vi "FTW-Logger-Construct.vi"(0 "Initialization Sequence":string, 5 "Logger Configuration":string, 11 "error in":errorcluster) -> (4 "FTW Logger":refnum<class "FTW-Logger-Instance.lvclass">, 6 "Incoming Requests":refnum<event-registration>, 15 "error out":errorcluster)   [LabVIEW 2013, in "FTW-Logger-Instance.lvclass"]
uses:
  FTW-Logger-Instance.lvclass
  request/FTW-Request.lvclass
  time/FTW-Time-DisplayFormat-Timestamp.ctl
  FTW-Logger-Instance.lvclass/FTW-Logger-Instance.ctl
  reflection/FTW-Reflection-Type.vi
  json/lib/FTW-JSON-Core-LibraryFilepath.vi
  json/lib/FTW-JSON-Core-GetFlattenedValue.vi
  json/lib/FTW-JSON-Core-LibraryError.vi
  json/FTW-JSON-Deserialize/FTW-JSON-Deserialize.xnode
panel:
  # "Inputs"
  # "Outputs"
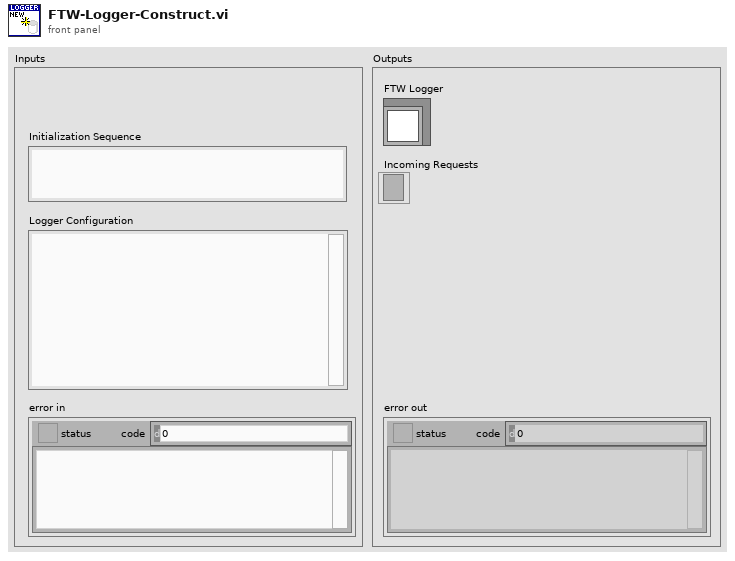
[diagram p1: front panel]
types:
  T1 = typedef "FTW-Time-DisplayFormat-Timestamp.ctl" = enum16{"YYYY-MM-DDT00:00:00.000Z (ISO-8601)", "YYYY-MM-DDT00-00-00Z (Simple ISO-8601)", "YYYY-MM-DD"}
  T2 = cluster{"LoggerDirectory":path, "LoggerDiskThrashDelay":u32, "LoggerName":string, "ApplicationName":string}
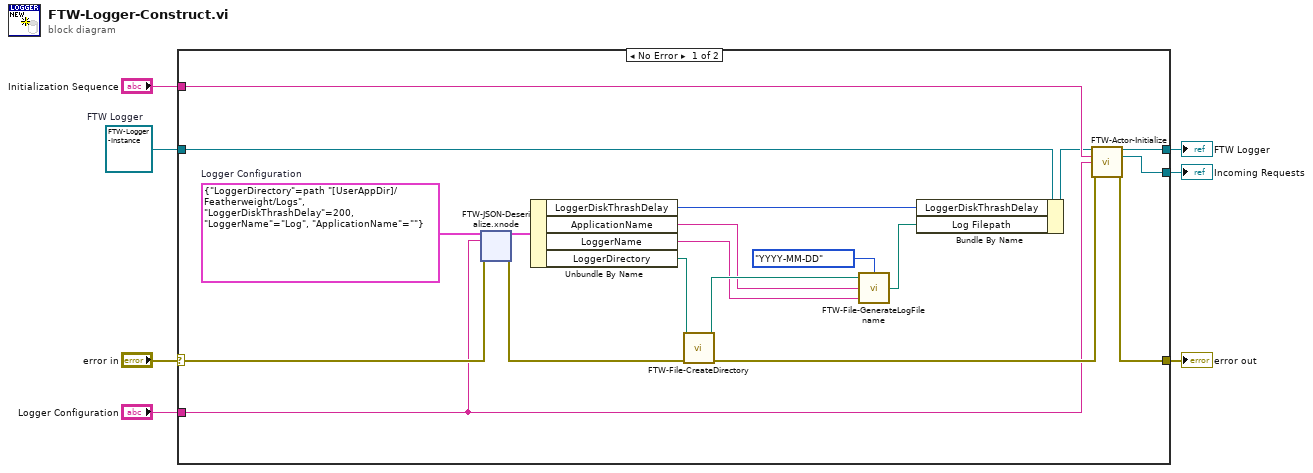
[diagram p0: block diagram]
diagram:
  w7 = refnum<class "FTW-Logger-Instance.lvclass"> refnum  # FTW Logger
  n1 = case shown="No Error" "error in" {
    selector: "error in" -> [w12 w62]
    tunnel: [w24 w62] -> w5
    tunnel: [w26 w61] -> w1
    tunnel: w7 -> [w22 w61]
    tunnel: "Logger Configuration" -> [w10 _]
    tunnel: [w25 _] -> w3
    tunnel: "Initialization Sequence" -> [w23 _]
    frame No Error {
      w9 = T2 {"LoggerDirectory"=path "[UserAppDir]/Featherweight/Logs", "LoggerDiskThrashDelay"=200, "LoggerName"="Log", "ApplicationName"=""}  # Logger Configuration
      n2 = xnode "FTW-JSON-Deserialize.xnode"("Type and Defaults"=w9, "JSON String"=w10, "error in"=w12) -> ("Values"=w8:T2, "error out"=w11:errorcluster)
      n3 = Unbundle By Name(w8) -> ("LoggerDiskThrashDelay"=w20:u32, "ApplicationName"=w17:string, "LoggerName"=w16:string, "LoggerDirectory"=w15:path)
      n4 = call "FTW-File-CreateDirectory.vi"("Directory to Create"=w15, "error in"=w11) -> ("Created Directory"=w18:path, "error out"=w13:errorcluster)  [unwired: 12 in]
      n5 = call "FTW-File-GenerateLogFilename.vi"("Date Format"=FTW-Time-DisplayFormat-Timestamp."YYYY-MM-DD", "Type"=w16, "Application"=w17, "Directory"=w18) -> ("Filepath"=w14:path)
      n6 = Bundle By Name(cluster=w22, "LoggerDiskThrashDelay"=w20, "Log Filepath"=w14) -> (w21:refnum<class "FTW-Logger-Instance.lvclass">)
      n7 = call-dynamic "FTW-Actor-Initialize.vi"("FTW Actor Instance Type"=w21, "Initialization Job Sequence"=w23, "Actor Instance Configuration"=w10, "error in"=w13) -> ("FTW Actor Instance"=w26:refnum<class "FTW-Logger-Instance.lvclass">, "Incoming Request"=w25:refnum<event-registration>, "error out"=w24:errorcluster)  [unwired: 9 in]
    }
    frame Error {
    }
  }
  "error out" <- w5
  "FTW Logger" <- w1
  "Incoming Requests" <- w3
